vi "p1.vi"() -> ()   [LabVIEW 2021, in "d18.lvlib"]
uses:
  d18.lvlib
  AOC/AOC.lvlib
panel:
  in  "Example":string
  in  "Example":bool
  out "Answer":u64
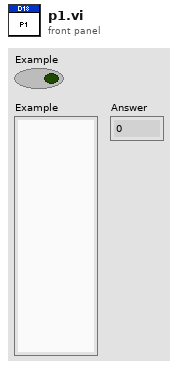
[diagram p1: front panel]
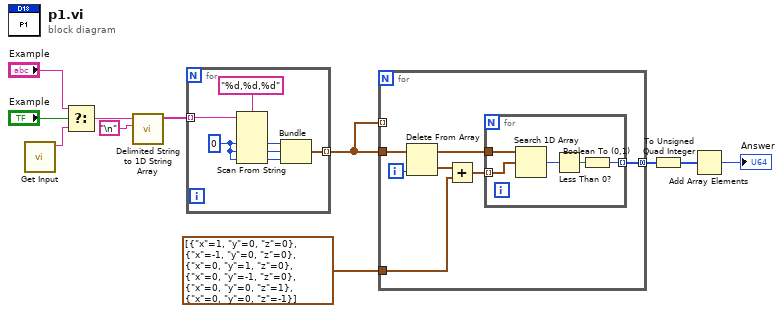
[diagram p0: block diagram]
diagram:
  n1 = call "Get Input.vi"() -> ("Input"=w11:string)  [unwired: 11 in]
  n2 = Select(t="Example", s="Example", f=w11) -> (s? t:f=w10:string)
  n3 = call <vilib>:"Delimited String to 1D String Array.vi"("delimiter"="\n", "delimited string"=w10) -> ("string array"=w6:string[])  [unwired: 9 in]
  n4 = for {
    tunnel: w6 -> [w18] mode=indexing
    tunnel: [w12] -> w5 mode=indexing
    w16 = i64 0
    n5 = Scan From String(format string="%d,%d,%d", input string=w18, default 1=w16, default 2=w16, default 3=w16) -> (output 1=w15:i64, output 2=w14:i64, output 3=w13:i64)  [unwired: 2 in, 3 out]
    n6 = Bundle(w15, w14, w13) -> (w12:cluster{i64, i64, i64})  [unwired: 1 in]
  }
  n7 = for {
    tunnel: w5 -> [_] mode=indexing
    tunnel: w5 -> [w25]
    tunnel: cluster{"x":i64, "y":i64, "z":i64}[] [{"x"=1, "y"=0, "z"=0}, {"x"=-1, "y"=0, "z"=0}, {"x"=0, "y"=1, "z"=0}, {"x"=0, "y"=-1, "z"=0}, {"x"=0, "y"=0, "z"=1}, {"x"=0, "y"=0, "z"=-1}] -> [w22]
    tunnel: [w19] -> w3 mode=concatenating
    i -> [w24]
    n8 = Delete From Array(array=w25, index=w24) -> (deleted portion=w23:cluster{i64, i64, i64}, array with subset deleted=w21:cluster{i64, i64, i64}[])  [unwired: 1 in]
    n9 = Add(x=w23, y=w22) -> (x+y=w20:cluster{i64, i64, i64}[])
    n10 = for {
      tunnel: w21 -> [w30]
      tunnel: w20 -> [w29] mode=indexing
      tunnel: [w26] -> w19 mode=indexing
      n11 = Search 1D Array(1D array=w30, element=w29) -> (index of element=w28:i32)  [unwired: 1 in]
      n12 = Less Than 0?(x=w28) -> (x < 0?=w27:bool)
      n13 = Boolean To (0,1)(Boolean=w27) -> (0, 1=w26:i16)
    }
  }
  n14 = To Unsigned Quad Integer(1:w3) -> (0:w1:u64[])
  n15 = Add Array Elements(numeric array=w1) -> (sum=→"Answer":u64)
